vi "LoopVI-V2 (Kenneth Goodenough's conflicted copy 2014-05-17).vi"() -> ()   [LabVIEW 2013]
uses:
  <vilib>/Utility/file.llb/Read From Spreadsheet File (DBL).vi
panel:
  in  "file path (dialog if empty)":path
  in  "Boolean":bool
  in  "measurement file\n\n         ??. txt":bool
  out "free gas model":cluster{"Y":dbl[], "Y":dbl[]}[](graph)
  in  "Fermi angle\n   (mrad)":dbl=7.0
  in  "stop 2":bool
  out "core electrons":cluster{"Y":dbl[], "Y":dbl[]}[](graph)
  in  "core width\n   (mrad)":dbl=5.0
  in  "fraction core\nannihilations":dbl=0.2 min=0.0 max=1.0 step=1e-05
  out "ZICHT  functie":cluster{"Y":dbl[], "Y":dbl[]}[](graph)
  in  "spleetbreedte\n      (mm)":dbl=1.0 min=0.1 max=5.0
  in  "collimator afstand\n       (mm)":dbl=500.0 min=100.0 max=1000.0
  in  "stop 4":bool
  out "XY Graph 4":cluster{ext[], "Array out":ext[]}[](graph)
  in  "alignment correction":dbl min=-10.0 max=10.0 step=0.0001
  in  "background \n coincidence counts":dbl min=0.0 max=100.0
  out "Fermi energy (eV)":dbl format="%#_3g"
  in  "22Na source radius (mm)":dbl=0.1 min=1e-05 max=3.0
  out "?":dbl format="%#_3g"
  in  "1d - Acar":bool caption="2d - Acar or DB"
  out "2d - Acar 2":bool
  out "2d - Acar 3":bool
  out "2d - Acar 4":bool
  out "XY Graph 5":cluster{ext[], "Array out":ext[]}[](graph)
  out "output cluster 2":cluster{ext[], ext[]}
  out "Sum of squared residuals":dbl
  in  "sigma (mrad) 2":dbl
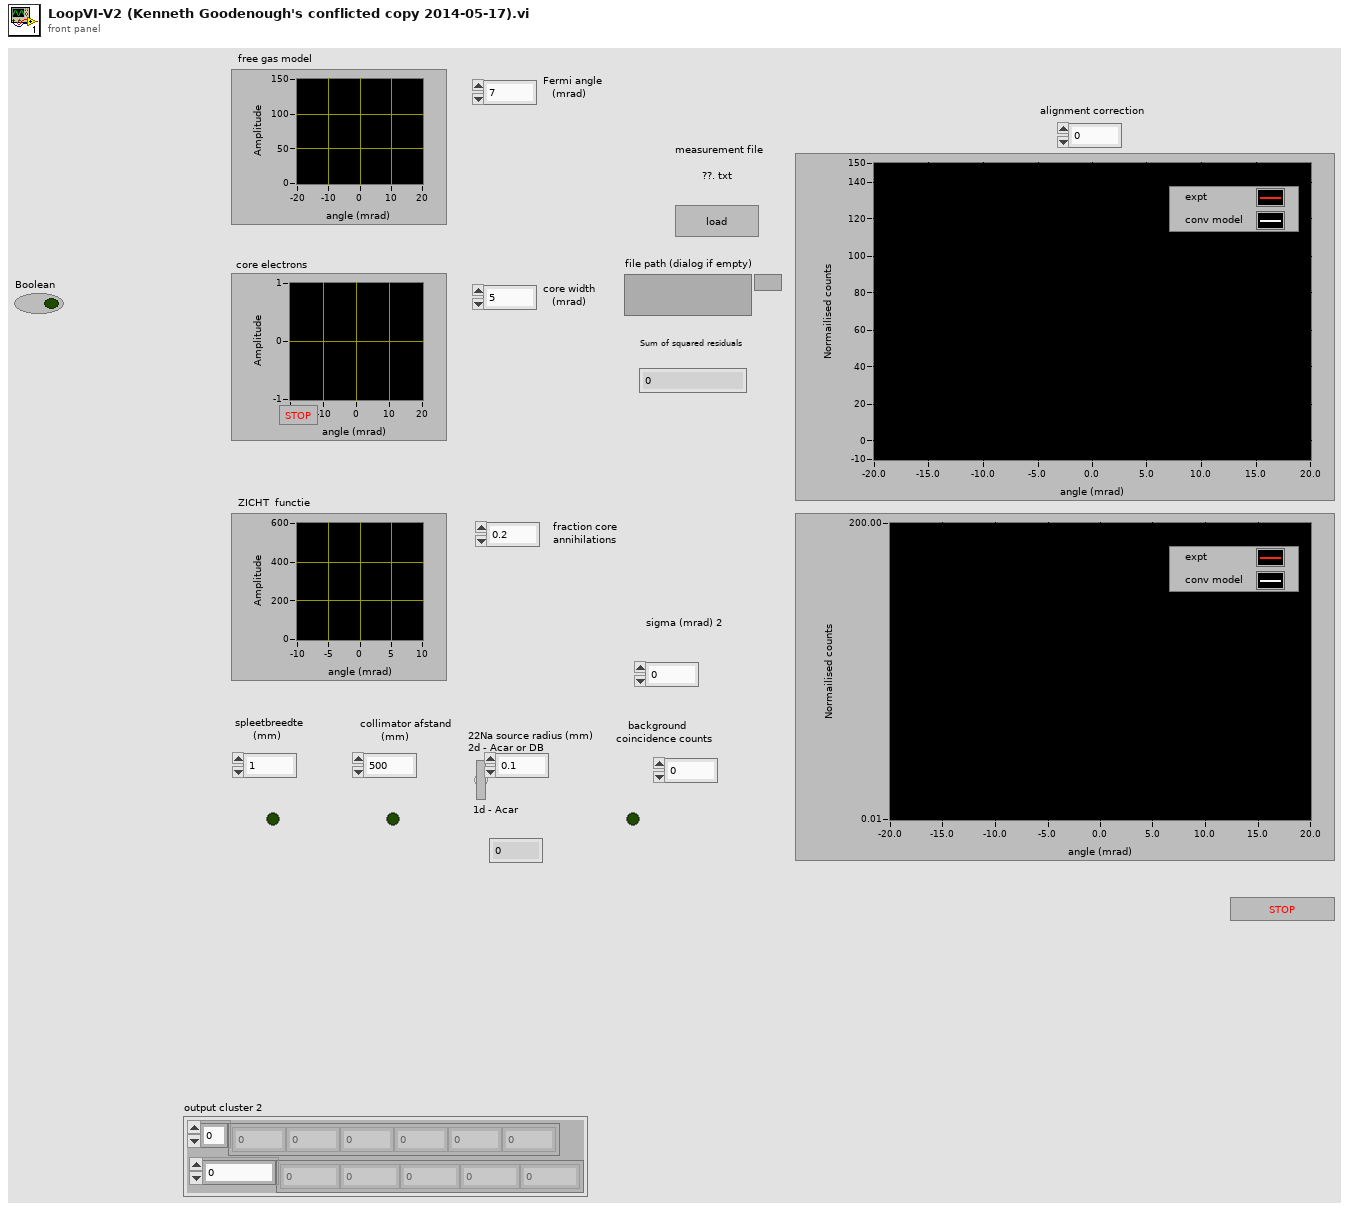
[diagram p1: front panel]
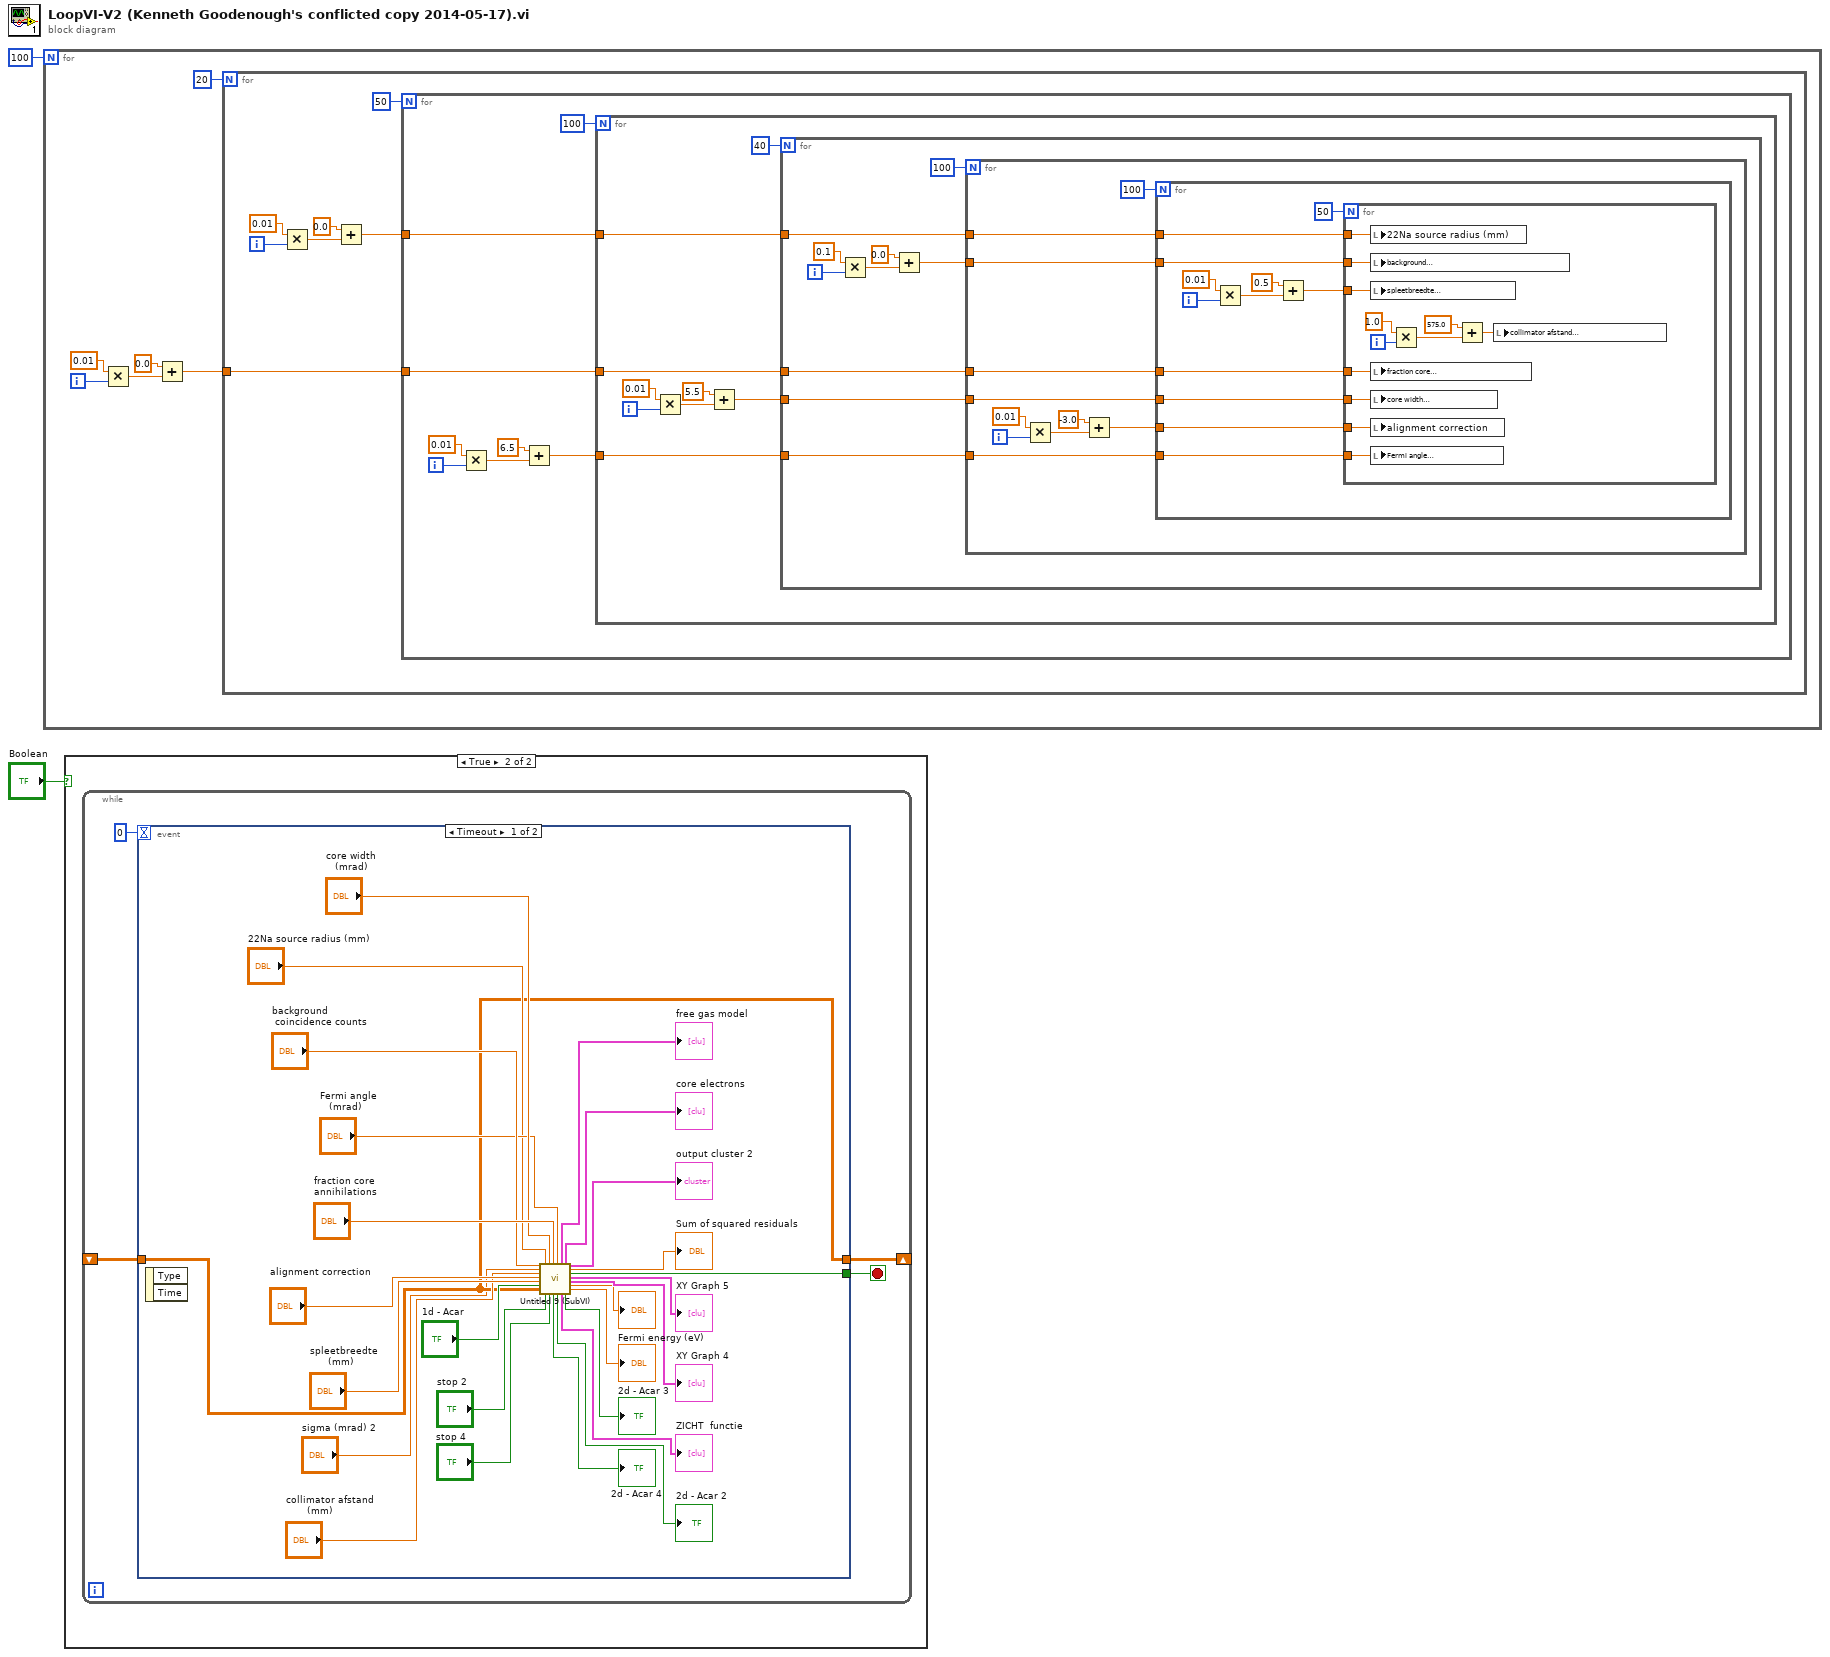
[diagram p0: block diagram]
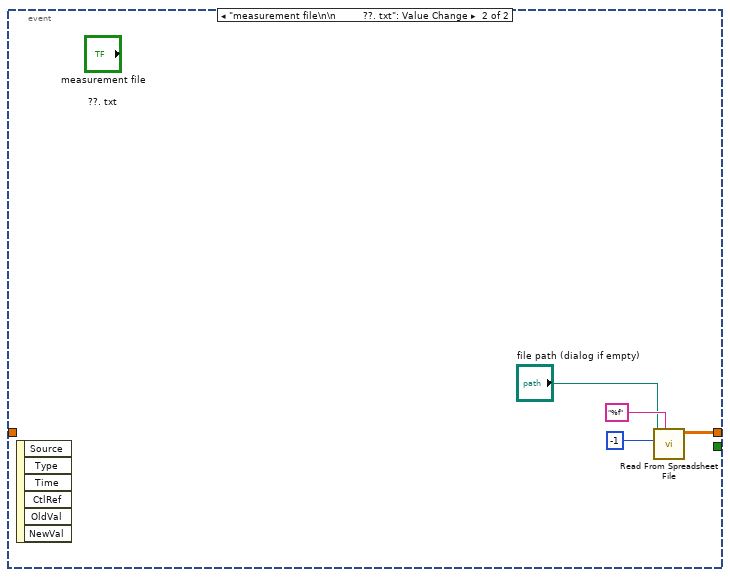
[diagram p3: hidden frame]
diagram:
  n1 = for {
    N: 100 -> [_]
    i -> [w8]
    n2 = Multiply(x=0.01, y=w8) -> (x*y=w6:dbl)
    n3 = Add(x=0.0, y=w6) -> (x+y=w4:dbl)
    n4 = for {
      N: 20 -> [_]
      tunnel: w4 -> [w10]
      i -> [w15]
      n5 = Multiply(x=0.01, y=w15) -> (x*y=w13:dbl)
      n6 = Add(x=0.0, y=w13) -> (x+y=w9:dbl)
      n7 = for {
        N: 50 -> [_]
        tunnel: w10 -> [w18]
        tunnel: w9 -> [w17]
        i -> [w23]
        n8 = Multiply(x=0.01, y=w23) -> (x*y=w21:dbl)
        n9 = Add(x=6.5, y=w21) -> (x+y=w16:dbl)
        n10 = for {
          N: 100 -> [_]
          tunnel: w18 -> [w24]
          tunnel: w17 -> [w25]
          tunnel: w16 -> [w26]
          i -> [w32]
          n11 = Multiply(x=0.01, y=w32) -> (x*y=w30:dbl)
          n12 = Add(x=5.5, y=w30) -> (x+y=w27:dbl)
          n13 = for {
            N: 40 -> [_]
            tunnel: w27 -> [w34]
            tunnel: w26 -> [w35]
            tunnel: w25 -> [w36]
            tunnel: w24 -> [w37]
            i -> [w42]
            n14 = Multiply(x=0.1, y=w42) -> (x*y=w40:dbl)
            n15 = Add(x=0.0, y=w40) -> (x+y=w33:dbl)
            n16 = for {
              N: 100 -> [_]
              tunnel: w37 -> [w48]
              tunnel: w36 -> [w47]
              tunnel: w35 -> [w46]
              tunnel: w34 -> [w45]
              tunnel: w33 -> [w44]
              i -> [w53]
              n17 = Multiply(x=0.01, y=w53) -> (x*y=w51:dbl)
              n18 = Add(x=-3.0, y=w51) -> (x+y=w43:dbl)
              n19 = for {
                N: 100 -> [_]
                tunnel: w48 -> [w59]
                tunnel: w47 -> [w58]
                tunnel: w46 -> [w57]
                tunnel: w45 -> [w56]
                tunnel: w44 -> [w55]
                tunnel: w43 -> [w54]
                i -> [w65]
                n20 = Multiply(x=0.01, y=w65) -> (x*y=w63:dbl)
                n21 = Add(x=0.5, y=w63) -> (x+y=w60:dbl)
                n22 = for {
                  N: 50 -> [_]
                  tunnel: w60 -> [w67]
                  tunnel: w59 -> [w73]
                  tunnel: w58 -> [w72]
                  tunnel: w57 -> [w71]
                  tunnel: w56 -> [w70]
                  tunnel: w55 -> [w69]
                  tunnel: w54 -> [w68]
                  i -> [w77]
                  n23 = local write "22Na source radius (mm)"(w72) -> ()
                  n24 = local write "background \n coincidence counts"(w69) -> ()
                  n25 = local write "spleetbreedte\n      (mm)"(w67) -> ()
                  n26 = local write "fraction core\nannihilations"(w73) -> ()
                  n27 = local write "core width\n   (mrad)"(w70) -> ()
                  n28 = local write "alignment correction"(w68) -> ()
                  n29 = local write "Fermi angle\n   (mrad)"(w71) -> ()
                  n30 = Multiply(x=1.0, y=w77) -> (x*y=w75:dbl)
                  n31 = Add(x=575.0, y=w75) -> (x+y=w66:dbl)
                  n32 = local write "collimator afstand\n       (mm)"(w66) -> ()
                }
              }
            }
          }
        }
      }
    }
  }
  n33 = case shown="True" "Boolean" {
    frame False {
    }
    frame True {
      n34 = while {
        shift-right: [w79] -> _
        shift-left: _ -> [w78]
        stop <- w81 stop-if-true
        n35 = event shown="[0] Timeout" {
          selector: _ -> [_ _]
          dyn-events: _ -> [_ _]
          timeout: 0 -> [_ _]
          tunnel: [w107 _] -> w81
          tunnel: [w97 w110] -> w79
          tunnel: w78 -> [w97 _]
          event Timeout {
            n36 = event-data() -> ()  [unwired: 1 in, 2 out]
            n37 = call "Untitled 9 (SubVI).vi"("background \n coincidence counts"="background \n coincidence counts", "sigma (mrad) in"="sigma (mrad) 2", "collimator afstand\n       (mm)"="collimator afstand\n       (mm)", "alignment correction"="alignment correction", "spleetbreedte\n      (mm)"="spleetbreedte\n      (mm)", "1d - Acar"="1d - Acar", "all rows"=w97, "22Na source radius (mm)"="22Na source radius (mm)", "stop in"="stop 2", "core width\n   (mrad)"="core width\n   (mrad)", "stop 4"="stop 4", "fraction core\nannihilations"="fraction core\nannihilations", "Fermi angle\n   (mrad)"="Fermi angle\n   (mrad)") -> ("2d - Acar 4"=→"2d - Acar 4":bool, "2d - Acar 2"=→"2d - Acar 2":bool, "free gas model"=→"free gas model":cluster{"Y":dbl[], "Y":dbl[]}[], "ZICHT  functie"=→"ZICHT  functie":cluster{"Y":dbl[], "Y":dbl[]}[], "core electrons"=→"core electrons":cluster{"Y":dbl[], "Y":dbl[]}[], "2d - Acar 3"=→"2d - Acar 3":bool, "output cluster 2"=→"output cluster 2":cluster{ext[], ext[]}, "Sum of squared residuals"=→"Sum of squared residuals":dbl, "stop 3"=w107:bool, "XY Graph 5"=→"XY Graph 5":cluster{ext[], "Array out":ext[]}[], "XY Graph 4"=→"XY Graph 4":cluster{ext[], "Array out":ext[]}[], 25:→"?":dbl, "Fermi energy (eV)"=→"Fermi energy (eV)":dbl)  [unwired: 2 in]
          }
          event "measurement file\n\n         ??. txt": Value Change {
            n38 = event-data() -> ()  [unwired: 1 in, 6 out]
            n39 = call-poly <vilib>:"Read From Spreadsheet File.vi"("format (%.3f)"="%f", "number of rows (all:-1)"=-1, "file path (dialog if empty)"="file path (dialog if empty)") -> ("all rows"=w110:ext[][])  [unwired: 4 in, 4 out]
          }
        }
      }
    }
  }
